vi "Main.vi"(7 "sweep rate, /min":dbl=0.2, 8 "sweep to:":dbl=-0.5, 9 "sweep":T6(radio)=enum."time_sweep") -> ()   [LabVIEW 2017] (continued)
                                n1009 = Number To Decimal String(number=w1251) -> (decimal integer string=w1250:string)  [unwired: 1 in]
                                n1010 = GPIB Write(0:w1250, 1:"OUTP?2") -> (6:w1256:errorcluster)  [unwired: 3 in, 1 out]
                                n1011 = GPIB Read(0:w1250, 1:3200, 3:w1256) -> (5:w1254:string)  [unwired: 2 in, 2 out]
                                n1012 = Fract/Exp String To Number(string=w1254) -> (number=w1253:dbl)  [unwired: 3 in, 1 out]
                                n1013 = Build Array (concatenate)(w1258, w1253) -> (w1257:dbl[])
                              }
                            }
                            n1014 = property on="data" class="Arr (strict)"("Value"=w1248) -> ()  [unwired: 2 in, 2 out]
                          }
                          frame #8 {
                            # "check if in-phase\nsignal on lock-in 5 \nis to be measured"
                            n1015 = property on="data" class="Arr (strict)"() -> ("Value"=w1260:dbl[])  [unwired: 2 in, 2 out]
                            n1016 = local read "SR830 5 ip"() -> (w1259:bool)
                            n1017 = case shown="True" w1259 {
                              tunnel: w1260 -> [w1262 w1271]
                              tunnel: [w1262 w1270] -> w1261
                              frame False {
                                # "we are not measuring in phase signal on lock-in 5 (SR830_5_ip)"
                              }
                              frame True {
                                # "we are  measuring lock-in 5 in phase (SR830_5_ip)"
                                n1018 = local read "SR830 5 addr"() -> (w1264:u8)
                                n1019 = Number To Decimal String(number=w1264) -> (decimal integer string=w1263:string)  [unwired: 1 in]
                                n1020 = GPIB Write(0:w1263, 1:"OUTP?1") -> (6:w1269:errorcluster)  [unwired: 3 in, 1 out]
                                n1021 = GPIB Read(0:w1263, 1:3200, 3:w1269) -> (5:w1267:string)  [unwired: 2 in, 2 out]
                                n1022 = Fract/Exp String To Number(string=w1267) -> (number=w1266:dbl)  [unwired: 3 in, 1 out]
                                n1023 = Build Array (concatenate)(w1271, w1266) -> (w1270:dbl[])
                              }
                            }
                            n1024 = property on="data" class="Arr (strict)"("Value"=w1261) -> ()  [unwired: 2 in, 2 out]
                          }
                          frame #9 {
                            # "check if out-of-phase\nsignal on lock-in 5 \nis to be measured"
                            n1025 = property on="data" class="Arr (strict)"() -> ("Value"=w1273:dbl[])  [unwired: 2 in, 2 out]
                            n1026 = local read "SR830 5 oop"() -> (w1272:bool)
                            n1027 = case shown="True" w1272 {
                              tunnel: w1273 -> [w1275 w1284]
                              tunnel: [w1275 w1283] -> w1274
                              frame False {
                                # "we are not measuring out of phase signal on lock-in 5 (SR830_5_oop)"
                              }
                              frame True {
                                # "we are  measuring lock-in 5 out of phase (SR830_5_oop)"
                                n1028 = local read "SR830 5 addr"() -> (w1277:u8)
                                n1029 = Number To Decimal String(number=w1277) -> (decimal integer string=w1276:string)  [unwired: 1 in]
                                n1030 = GPIB Write(0:w1276, 1:"OUTP?2") -> (6:w1282:errorcluster)  [unwired: 3 in, 1 out]
                                n1031 = GPIB Read(0:w1276, 1:3200, 3:w1282) -> (5:w1280:string)  [unwired: 2 in, 2 out]
                                n1032 = Fract/Exp String To Number(string=w1280) -> (number=w1279:dbl)  [unwired: 3 in, 1 out]
                                n1033 = Build Array (concatenate)(w1284, w1279) -> (w1283:dbl[])
                              }
                            }
                            n1034 = property on="data" class="Arr (strict)"("Value"=w1274) -> ()  [unwired: 2 in, 2 out]
                          }
                          frame #10 {
                            # "check if in-phase\nsignal on lock-in 6 \nis to be measured"
                            n1035 = property on="data" class="Arr (strict)"() -> ("Value"=w1286:dbl[])  [unwired: 2 in, 2 out]
                            n1036 = local read "SR830_6_ip"() -> (w1285:bool)
                            n1037 = case shown="True" w1285 {
                              tunnel: w1286 -> [w1288 w1297]
                              tunnel: [w1288 w1296] -> w1287
                              frame False {
                                # "we are not measuring in phase signal on lock-in 6 (SR830_6_ip)"
                              }
                              frame True {
                                # "we are  measuring lock-in 6 in phase (SR830_6_ip)"
                                n1038 = local read "SR830_6"() -> (w1290:u8)
                                n1039 = Number To Decimal String(number=w1290) -> (decimal integer string=w1289:string)  [unwired: 1 in]
                                n1040 = GPIB Write(0:w1289, 1:"OUTR?1") -> (6:w1295:errorcluster)  [unwired: 3 in, 1 out]
                                n1041 = GPIB Read(0:w1289, 1:3200, 3:w1295) -> (5:w1293:string)  [unwired: 2 in, 2 out]
                                n1042 = Fract/Exp String To Number(string=w1293) -> (number=w1292:dbl)  [unwired: 3 in, 1 out]
                                n1043 = Build Array (concatenate)(w1297, w1292) -> (w1296:dbl[])
                              }
                            }
                            n1044 = property on="data" class="Arr (strict)"("Value"=w1287) -> ()  [unwired: 2 in, 2 out]
                          }
                          frame #11 {
                            # "check if out-of-phase\nsignal on lock-in 6 \nis to be measured"
                            n1045 = property on="data" class="Arr (strict)"() -> ("Value"=w1299:dbl[])  [unwired: 2 in, 2 out]
                            n1046 = local read "SR830_6_oop"() -> (w1298:bool)
                            n1047 = case shown="True" w1298 {
                              tunnel: w1299 -> [w1301 w1310]
                              tunnel: [w1301 w1309] -> w1300
                              frame False {
                                # "we are not measuring out of phase signal on lock-in 6 (SR830_6_oop)"
                              }
                              frame True {
                                # "we are  measuring lock-in 6, out of phase (SR830_6_oop)"
                                n1048 = local read "SR830_6"() -> (w1303:u8)
                                n1049 = Number To Decimal String(number=w1303) -> (decimal integer string=w1302:string)  [unwired: 1 in]
                                n1050 = GPIB Write(0:w1302, 1:"OUTR?2") -> (6:w1308:errorcluster)  [unwired: 3 in, 1 out]
                                n1051 = GPIB Read(0:w1302, 1:3200, 3:w1308) -> (5:w1306:string)  [unwired: 2 in, 2 out]
                                n1052 = Fract/Exp String To Number(string=w1306) -> (number=w1305:dbl)  [unwired: 3 in, 1 out]
                                n1053 = Build Array (concatenate)(w1310, w1305) -> (w1309:dbl[])
                              }
                            }
                            n1054 = property on="data" class="Arr (strict)"("Value"=w1300) -> ()  [unwired: 2 in, 2 out]
                          }
                          frame #12 {
                            # "check if in-phase\nsignal on lock-in 7 \nis to be measured"
                            n1055 = property on="data" class="Arr (strict)"() -> ("Value"=w1312:dbl[])  [unwired: 2 in, 2 out]
                            n1056 = local read "SR830_7_ip"() -> (w1311:bool)
                            n1057 = case shown="True" w1311 {
                              tunnel: w1312 -> [w1314 w1323]
                              tunnel: [w1314 w1322] -> w1313
                              frame False {
                              }
                              frame True {
                                # "we are  measuring lock-in 7 in phase (SR830_7_ip)"
                                n1058 = local read "SR830_7"() -> (w1316:u8)
                                n1059 = Number To Decimal String(number=w1316) -> (decimal integer string=w1315:string)  [unwired: 1 in]
                                n1060 = GPIB Write(0:w1315, 1:"OUTR?1") -> (6:w1321:errorcluster)  [unwired: 3 in, 1 out]
                                n1061 = GPIB Read(0:w1315, 1:3200, 3:w1321) -> (5:w1319:string)  [unwired: 2 in, 2 out]
                                n1062 = Fract/Exp String To Number(string=w1319) -> (number=w1318:dbl)  [unwired: 3 in, 1 out]
                                n1063 = Build Array (concatenate)(w1323, w1318) -> (w1322:dbl[])
                              }
                            }
                            n1064 = property on="data" class="Arr (strict)"("Value"=w1313) -> ()  [unwired: 2 in, 2 out]
                          }
                          frame #13 {
                            # "check if out-of-phase\nsignal on lock-in 7 \nis to be measured"
                            n1065 = property on="data" class="Arr (strict)"() -> ("Value"=w1325:dbl[])  [unwired: 2 in, 2 out]
                            n1066 = local read "SR830_7_oop"() -> (w1324:bool)
                            n1067 = case shown="True" w1324 {
                              tunnel: w1325 -> [w1327 w1336]
                              tunnel: [w1327 w1335] -> w1326
                              frame False {
                              }
                              frame True {
                                # "we are  measuring lock-in 7 out of phase (SR830_7_oop)"
                                n1068 = local read "SR830_7"() -> (w1329:u8)
                                n1069 = Number To Decimal String(number=w1329) -> (decimal integer string=w1328:string)  [unwired: 1 in]
                                n1070 = GPIB Write(0:w1328, 1:"OUTR?2") -> (6:w1334:errorcluster)  [unwired: 3 in, 1 out]
                                n1071 = GPIB Read(0:w1328, 1:3200, 3:w1334) -> (5:w1332:string)  [unwired: 2 in, 2 out]
                                n1072 = Fract/Exp String To Number(string=w1332) -> (number=w1331:dbl)  [unwired: 3 in, 1 out]
                                n1073 = Build Array (concatenate)(w1336, w1331) -> (w1335:dbl[])
                              }
                            }
                            n1074 = property on="data" class="Arr (strict)"("Value"=w1326) -> ()  [unwired: 2 in, 2 out]
                          }
                          frame #14 {
                            # "check if in-phase\nsignal on lock-in 8 \nis to be measured"
                            n1075 = property on="data" class="Arr (strict)"() -> ("Value"=w1338:dbl[])  [unwired: 2 in, 2 out]
                            n1076 = local read "SR830_8_ip"() -> (w1337:bool)
                            n1077 = case shown="True" w1337 {
                              tunnel: w1338 -> [w1340 w1349]
                              tunnel: [w1340 w1348] -> w1339
                              frame False {
                              }
                              frame True {
                                # "we are  measuring lock-in 8 in phase (SR830_8_ip)"
                                n1078 = local read "SR830_8"() -> (w1342:u8)
                                n1079 = Number To Decimal String(number=w1342) -> (decimal integer string=w1341:string)  [unwired: 1 in]
                                n1080 = GPIB Write(0:w1341, 1:"OUTR?1") -> (6:w1347:errorcluster)  [unwired: 3 in, 1 out]
                                n1081 = GPIB Read(0:w1341, 1:3200, 3:w1347) -> (5:w1345:string)  [unwired: 2 in, 2 out]
                                n1082 = Fract/Exp String To Number(string=w1345) -> (number=w1344:dbl)  [unwired: 3 in, 1 out]
                                n1083 = Build Array (concatenate)(w1349, w1344) -> (w1348:dbl[])
                              }
                            }
                            n1084 = property on="data" class="Arr (strict)"("Value"=w1339) -> ()  [unwired: 2 in, 2 out]
                          }
                          frame #15 {
                            # "check if out-of-phase\nsignal on lock-in 8 \nis to be measured"
                            n1085 = property on="data" class="Arr (strict)"() -> ("Value"=w1351:dbl[])  [unwired: 2 in, 2 out]
                            n1086 = local read "SR830_8_oop"() -> (w1350:bool)
                            n1087 = case shown="True" w1350 {
                              tunnel: w1351 -> [w1353 w1362]
                              tunnel: [w1353 w1361] -> w1352
                              frame False {
                              }
                              frame True {
                                # "we are  measuring lock-in 8 out of phase (SR830_8_oop)"
                                n1088 = local read "SR830_8"() -> (w1355:u8)
                                n1089 = Number To Decimal String(number=w1355) -> (decimal integer string=w1354:string)  [unwired: 1 in]
                                n1090 = GPIB Write(0:w1354, 1:"OUTR?2") -> (6:w1360:errorcluster)  [unwired: 3 in, 1 out]
                                n1091 = GPIB Read(0:w1354, 1:3200, 3:w1360) -> (5:w1358:string)  [unwired: 2 in, 2 out]
                                n1092 = Fract/Exp String To Number(string=w1358) -> (number=w1357:dbl)  [unwired: 3 in, 1 out]
                                n1093 = Build Array (concatenate)(w1362, w1357) -> (w1361:dbl[])
                              }
                            }
                            n1094 = property on="data" class="Arr (strict)"("Value"=w1352) -> ()  [unwired: 2 in, 2 out]
                          }
                          frame #16 {
                            # "Measure MFLI_V if \nit is checked"
                            n1095 = property on="MFLI_V1" class="Bool (strict)"() -> ("Value"=w1363:bool)  [unwired: 2 in, 2 out]
                            n1096 = property on="data" class="Arr (strict)"() -> ("Value"=w1365:dbl[])  [unwired: 2 in, 2 out]
                            n1097 = case shown="True" w1363 {
                              tunnel: w1365 -> [w1366 w1371]
                              tunnel: [w1366 w1370] -> w1364
                              frame False {
                                # "We are not recording Step Value if it is linetrace"
                              }
                              frame True {
                                n1098 = flat-sequence {
                                tunnel: [w1375] -> w1369
                                tunnel: [w1374] -> w1368
                                tunnel: [w1373] -> w1367
                                frame #0 {
                                n1099 = property on="HandleOut" class="Clust (strict)"() -> ("Value"=w1377:T5)  [unwired: 2 in, 2 out]
                                n1100 = call "MFLIcontrol.vi"("MFLI function"=MFLIcommand."measure XY on demod0", "handle in"=w1377) -> ("Demod Sample Out 2"=w1372:T22)  [unwired: 6 in, 3 out]
                                n1101 = Unbundle(w1372) -> ("X (Vrms)"=w1375:dbl, "Y (Vrms)"=w1374:dbl, "Freq (Hz)"=w1373:dbl)  [unwired: 6 out]
                                }
                                }
                                n1102 = Build Array (concatenate)(w1371, w1369, w1368, w1367) -> (w1370:dbl[])
                              }
                            }
                            n1103 = property on="data" class="Arr (strict)"("Value"=w1364) -> ()  [unwired: 2 in, 2 out]
                          }
                          frame #17 {
                            # "Measure MFLI_I if \nit is checked"
                            n1104 = property on="MFLI_I1" class="Bool (strict)"() -> ("Value"=w1378:bool)  [unwired: 2 in, 2 out]
                            n1105 = property on="data" class="Arr (strict)"() -> ("Value"=w1380:dbl[])  [unwired: 2 in, 2 out]
                            n1106 = case shown="True" w1378 {
                              tunnel: w1380 -> [w1381 w1386]
                              tunnel: [w1381 w1385] -> w1379
                              frame False {
                                # "We are not recording Step Value if it is linetrace"
                              }
                              frame True {
                                n1107 = flat-sequence {
                                tunnel: [w1389] -> w1384
                                tunnel: [w1388] -> w1383
                                tunnel: [w1387] -> w1382
                                frame #0 {
                                n1108 = property on="HandleOut" class="Clust (strict)"() -> ("Value"=w1392:T5)  [unwired: 2 in, 2 out]
                                n1109 = call "MFLIcontrol.vi"("MFLI function"=MFLIcommand."measure current", "handle in"=w1392) -> ("Demod Sample Out 3"=w1390:T22)  [unwired: 6 in, 3 out]
                                n1110 = Unbundle(w1390) -> ("X (Vrms)"=w1389:dbl, "Y (Vrms)"=w1388:dbl, "Freq (Hz)"=w1387:dbl)  [unwired: 6 out]
                                }
                                }
                                n1111 = Build Array (concatenate)(w1386, w1384, w1383, w1382) -> (w1385:dbl[])
                              }
                            }
                            n1112 = property on="data" class="Arr (strict)"("Value"=w1379) -> ()  [unwired: 2 in, 2 out]
                          }
                          frame #18 {
                            # "Measure MFLI_V if \nit is checked"
                            n1113 = local read "MFLI_V2"() -> (w1393:bool)
                            n1114 = property on="data" class="Arr (strict)"() -> ("Value"=w1395:dbl[])  [unwired: 2 in, 2 out]
                            n1115 = case shown="True" w1393 {
                              tunnel: w1395 -> [w1396 w1401]
                              tunnel: [w1396 w1400] -> w1394
                              frame False {
                              }
                              frame True {
                                n1116 = flat-sequence {
                                tunnel: [w1406] -> w1399
                                tunnel: [w1405] -> w1398
                                tunnel: [w1404] -> w1397
                                frame #0 {
                                n1117 = property on="Handle Out 2" class="Clust (strict)"() -> ("Value"=w1402:T5)  [unwired: 2 in, 2 out]
                                n1118 = call "MFLIcontrol.vi"("MFLI function"=MFLIcommand."measure XY on demod0", "handle in"=w1402) -> ("Demod Sample Out 2"=w1403:T22)  [unwired: 6 in, 3 out]
                                n1119 = Unbundle(w1403) -> ("X (Vrms)"=w1406:dbl, "Y (Vrms)"=w1405:dbl, "Freq (Hz)"=w1404:dbl)  [unwired: 6 out]
                                }
                                }
                                n1120 = Build Array (concatenate)(w1401, w1399, w1398, w1397) -> (w1400:dbl[])
                              }
                            }
                            n1121 = property on="data" class="Arr (strict)"("Value"=w1394) -> ()  [unwired: 2 in, 2 out]
                          }
                          frame #19 {
                            # "Measure MFLI_I if \nit is checked"
                            n1122 = local read "MFLI_I2"() -> (w1408:bool)
                            n1123 = property on="data" class="Arr (strict)"() -> ("Value"=w1410:dbl[])  [unwired: 2 in, 2 out]
                            n1124 = case shown="True" w1408 {
                              tunnel: w1410 -> [w1411 w1416]
                              tunnel: [w1411 w1415] -> w1409
                              frame False {
                              }
                              frame True {
                                n1125 = flat-sequence {
                                tunnel: [w1421] -> w1414
                                tunnel: [w1420] -> w1413
                                tunnel: [w1419] -> w1412
                                frame #0 {
                                n1126 = property on="Handle Out 2" class="Clust (strict)"() -> ("Value"=w1418:T5)  [unwired: 2 in, 2 out]
                                n1127 = call "MFLIcontrol.vi"("MFLI function"=MFLIcommand."measure current", "handle in"=w1418) -> ("Demod Sample Out 3"=w1417:T22)  [unwired: 6 in, 3 out]
                                n1128 = Unbundle(w1417) -> ("X (Vrms)"=w1421:dbl, "Y (Vrms)"=w1420:dbl, "Freq (Hz)"=w1419:dbl)  [unwired: 6 out]
                                }
                                }
                                n1129 = Build Array (concatenate)(w1416, w1414, w1413, w1412) -> (w1415:dbl[])
                              }
                            }
                            n1130 = property on="data" class="Arr (strict)"("Value"=w1409) -> ()  [unwired: 2 in, 2 out]
                          }
                          frame #20 {
                            # "check if voltage \non 2400 SouceMeter 1\nis to be measured"
                            n1131 = property on="data" class="Arr (strict)"() -> ("Value"=w1424:dbl[])  [unwired: 2 in, 2 out]
                            n1132 = local read "2400 1 meas v"() -> (w1423:bool)
                            n1133 = case shown="True" w1423 {
                              tunnel: w1424 -> [w1426 w1437]
                              tunnel: [w1426 w1436] -> w1425
                              frame False {
                                # "we are not measuring 2400 1, voltage (2400_1_v)"
                              }
                              frame True {
                                # "we are  measuring 2400 1, voltage (2400_1_v)"
                                n1134 = local read "2400 1 addr"() -> (w1431:u8)
                                n1135 = Number To Decimal String(number=w1431) -> (decimal integer string=w1430:string)  [unwired: 1 in]
                                n1136 = GPIB Write(0:w1430, 1:":READ?") -> (6:w1435:errorcluster)  [unwired: 3 in, 1 out]
                                n1137 = GPIB Read(0:w1430, 1:3200, 3:w1435) -> (5:w1428:string)  [unwired: 2 in, 2 out]
                                n1138 = String Subset(string=w1428, length (rest)=13) -> (substring=w1427:string)  [unwired: 1 in]
                                n1139 = Fract/Exp String To Number(string=w1427) -> (number=w1433:dbl)  [unwired: 3 in, 1 out]
                                n1140 = Build Array (concatenate)(w1437, w1433) -> (w1436:dbl[])
                              }
                            }
                            n1141 = property on="data" class="Arr (strict)"("Value"=w1425) -> ()  [unwired: 2 in, 2 out]
                          }
                          frame #21 {
                            # "check if current \non 2400 SouceMeter 1\nis to be measured"
                            n1142 = property on="data" class="Arr (strict)"() -> ("Value"=w1439:dbl[])  [unwired: 2 in, 2 out]
                            n1143 = local read "2400 1 meas i"() -> (w1438:bool)
                            n1144 = case shown="True" w1438 {
                              tunnel: w1439 -> [w1441 w1453]
                              tunnel: [w1441 w1452] -> w1440
                              frame False {
                                # "we are not measuring 2400 1, current (2400_1_i)"
                              }
                              frame True {
                                # "we are  measuring 2400 1, current (2400_1_i)"
                                n1145 = local read "2400 1 addr"() -> (w1447:u8)
                                n1146 = Number To Decimal String(number=w1447) -> (decimal integer string=w1446:string)  [unwired: 1 in]
                                n1147 = GPIB Write(0:w1446, 1:":READ?") -> (6:w1451:errorcluster)  [unwired: 3 in, 1 out]
                                n1148 = GPIB Read(0:w1446, 1:3200, 3:w1451) -> (5:w1444:string)  [unwired: 2 in, 2 out]
                                n1149 = String Subset(string=w1444, offset (0)=14, length (rest)=13) -> (substring=w1443:string)
                                n1150 = Fract/Exp String To Number(string=w1443) -> (number=w1449:dbl)  [unwired: 3 in, 1 out]
                                n1151 = Build Array (concatenate)(w1453, w1449) -> (w1452:dbl[])
                              }
                            }
                            n1152 = property on="data" class="Arr (strict)"("Value"=w1440) -> ()  [unwired: 2 in, 2 out]
                          }
                          frame #22 {
                            # "check if voltage \non 2400 SouceMeter 2\nis to be measured"
                            n1153 = property on="data" class="Arr (strict)"() -> ("Value"=w1455:dbl[])  [unwired: 2 in, 2 out]
                            n1154 = local read "2400 2 meas v"() -> (w1454:bool)
                            n1155 = case shown="True" w1454 {
                              tunnel: w1455 -> [w1457 w1468]
                              tunnel: [w1457 w1467] -> w1456
                              frame False {
                                # "we are not measuring 2400 2, voltage (2400_2_v)"
                              }
                              frame True {
                                # "we are  measuring 2400 2, voltage (2400_2_v)"
                                n1156 = local read "2400 2 addr"() -> (w1462:u8)
                                n1157 = Number To Decimal String(number=w1462) -> (decimal integer string=w1461:string)  [unwired: 1 in]
                                n1158 = GPIB Write(0:w1461, 1:":READ?") -> (6:w1466:errorcluster)  [unwired: 3 in, 1 out]
                                n1159 = GPIB Read(0:w1461, 1:3200, 3:w1466) -> (5:w1459:string)  [unwired: 2 in, 2 out]
                                n1160 = String Subset(string=w1459, length (rest)=13) -> (substring=w1458:string)  [unwired: 1 in]
                                n1161 = Fract/Exp String To Number(string=w1458) -> (number=w1464:dbl)  [unwired: 3 in, 1 out]
                                n1162 = Build Array (concatenate)(w1468, w1464) -> (w1467:dbl[])
                              }
                            }
                            n1163 = property on="data" class="Arr (strict)"("Value"=w1456) -> ()  [unwired: 2 in, 2 out]
                          }
                          frame #23 {
                            # "check if current \non 2400 SouceMeter 2\nis to be measured"
                            n1164 = property on="data" class="Arr (strict)"() -> ("Value"=w1470:dbl[])  [unwired: 2 in, 2 out]
                            n1165 = local read "2400 2 meas i"() -> (w1469:bool)
                            n1166 = case shown="True" w1469 {
                              tunnel: w1470 -> [w1472 w1484]
                              tunnel: [w1472 w1483] -> w1471
                              frame False {
                                # "we are not measuring 2400 2, current (2400_2_i)"
                              }
                              frame True {
                                # "we are  measuring 2400 2, current (2400_2_i)"
                                n1167 = local read "2400 2 addr"() -> (w1478:u8)
                                n1168 = Number To Decimal String(number=w1478) -> (decimal integer string=w1477:string)  [unwired: 1 in]
                                n1169 = GPIB Write(0:w1477, 1:":READ?") -> (6:w1482:errorcluster)  [unwired: 3 in, 1 out]
                                n1170 = GPIB Read(0:w1477, 1:3200, 3:w1482) -> (5:w1475:string)  [unwired: 2 in, 2 out]
                                n1171 = String Subset(string=w1475, offset (0)=14, length (rest)=13) -> (substring=w1474:string)
                                n1172 = Fract/Exp String To Number(string=w1474) -> (number=w1480:dbl)  [unwired: 3 in, 1 out]
                                n1173 = Build Array (concatenate)(w1484, w1480) -> (w1483:dbl[])
                              }
                            }
                            n1174 = property on="data" class="Arr (strict)"("Value"=w1471) -> ()  [unwired: 2 in, 2 out]
                          }
                          frame #24 {
                            # "check if voltage \non 2400 SouceMeter 3\nis to be measured"
                            n1175 = property on="data" class="Arr (strict)"() -> ("Value"=w1486:dbl[])  [unwired: 2 in, 2 out]
                            n1176 = local read "2400 3 meas v"() -> (w1485:bool)
                            n1177 = case shown="True" w1485 {
                              tunnel: w1486 -> [w1488 w1499]
                              tunnel: [w1488 w1498] -> w1487
                              frame False {
                                # "we are not measuring 2400 3, voltage (2400_3_v)"
                              }
                              frame True {
                                # "we are  measuring 2400 3, voltage (2400_3_v)"
                                n1178 = local read "2400 3 addr"() -> (w1493:u8)
                                n1179 = Number To Decimal String(number=w1493) -> (decimal integer string=w1492:string)  [unwired: 1 in]
                                n1180 = GPIB Write(0:w1492, 1:":READ?") -> (6:w1497:errorcluster)  [unwired: 3 in, 1 out]
                                n1181 = GPIB Read(0:w1492, 1:3200, 3:w1497) -> (5:w1490:string)  [unwired: 2 in, 2 out]
                                n1182 = String Subset(string=w1490, length (rest)=13) -> (substring=w1489:string)  [unwired: 1 in]
                                n1183 = Fract/Exp String To Number(string=w1489) -> (number=w1495:dbl)  [unwired: 3 in, 1 out]
                                n1184 = Build Array (concatenate)(w1499, w1495) -> (w1498:dbl[])
                              }
                            }
                            n1185 = property on="data" class="Arr (strict)"("Value"=w1487) -> ()  [unwired: 2 in, 2 out]
                          }
                          frame #25 {
                            # "check if current \non 2400 SouceMeter 3\nis to be measured"
                            n1186 = property on="data" class="Arr (strict)"() -> ("Value"=w1501:dbl[])  [unwired: 2 in, 2 out]
                            n1187 = local read "2400 3 meas i"() -> (w1500:bool)
                            n1188 = case shown="True" w1500 {
                              tunnel: w1501 -> [w1503 w1515]
                              tunnel: [w1503 w1514] -> w1502
                              frame False {
                                # "we are not measuring 2400 3, current (2400_3_i)"
                              }
                              frame True {
                                # "we are  measuring 2400 3, current (2400_3_i)"
                                n1189 = local read "2400 3 addr"() -> (w1509:u8)
                                n1190 = Number To Decimal String(number=w1509) -> (decimal integer string=w1508:string)  [unwired: 1 in]
                                n1191 = GPIB Write(0:w1508, 1:":READ?") -> (6:w1513:errorcluster)  [unwired: 3 in, 1 out]
                                n1192 = GPIB Read(0:w1508, 1:3200, 3:w1513) -> (5:w1506:string)  [unwired: 2 in, 2 out]
                                n1193 = String Subset(string=w1506, offset (0)=14, length (rest)=13) -> (substring=w1505:string)
                                n1194 = Fract/Exp String To Number(string=w1505) -> (number=w1511:dbl)  [unwired: 3 in, 1 out]
                                n1195 = Build Array (concatenate)(w1515, w1511) -> (w1514:dbl[])
                              }
                            }
                            n1196 = property on="data" class="Arr (strict)"("Value"=w1502) -> ()  [unwired: 2 in, 2 out]
                          }
                          frame #26 {
                            # "check if 1st channel \non Keithley 2182A 1\nis to be measured"
                            n1197 = property on="data" class="Arr (strict)"() -> ("Value"=w1517:dbl[])  [unwired: 2 in, 2 out]
                            n1198 = local read "2182A 1 ch1"() -> (w1516:bool)
                            n1199 = case shown="True" w1516 {
                              tunnel: w1517 -> [w1519 w1528]
                              tunnel: [w1519 w1527] -> w1518
                              frame False {
                                # "we are not measuring 2182A 1 channel 1 (2182A_1_ch1)"
                              }
                              frame True {
                                # "we are  measuring 2182A 1 channel 1 (2182A_1_ch1)"
                                n1200 = local read "2182A 1 addr"() -> (w1522:u8)
                                n1201 = Number To Decimal String(number=w1522) -> (decimal integer string=w1521:string)  [unwired: 1 in]
                                n1202 = GPIB Write(0:w1521, 1:":SENSe:DATA:FRES?") -> (6:w1526:errorcluster)  [unwired: 3 in, 1 out]
                                n1203 = GPIB Read(0:w1521, 1:200, 3:w1526) -> (5:w1520:string)  [unwired: 2 in, 2 out]
                                n1204 = Fract/Exp String To Number(string=w1520) -> (number=w1524:dbl)  [unwired: 3 in, 1 out]
                                n1205 = Build Array (concatenate)(w1528, w1524) -> (w1527:dbl[])
                              }
                            }
                            n1206 = property on="data" class="Arr (strict)"("Value"=w1518) -> ()  [unwired: 2 in, 2 out]
                          }
                          frame #27 {
                            # "check if 2nd channel \non Keithley 2182A 1\nis to be measured"
                            n1207 = property on="data" class="Arr (strict)"() -> ("Value"=w1530:dbl[])  [unwired: 2 in, 2 out]
                            n1208 = local read "2182A 1 ch2"() -> (w1529:bool)
                            n1209 = case shown="True" w1529 {
                              tunnel: w1530 -> [w1532 w1545]
                              tunnel: [w1532 w1544] -> w1531
                              frame False {
                                # "we are not measuring 2182A 1 channel 2 (2182A_1_ch2)"
                              }
                              frame True {
                                # "switching to channel 2 and then\nback to channel 1"
                                # "we are  measuring 2182A 1 channel 2 (2182A_1_ch2)"
                                n1210 = local read "2182A 1 addr"() -> (w1539:u8)
                                n1211 = Number To Decimal String(number=w1539) -> (decimal integer string=w1534:string)  [unwired: 1 in]
                                n1212 = GPIB Write(0:w1534, 1:":SENSe:CHAN 2") -> (6:w1536:errorcluster)  [unwired: 3 in, 1 out]
                                n1213 = GPIB Write(0:w1534, 1:":SENSe:DATA:FRES?", 3:w1536) -> (6:w1543:errorcluster)  [unwired: 2 in, 1 out]
                                n1214 = GPIB Read(0:w1534, 1:200, 3:w1543) -> (5:w1538:string, 7:w1535:errorcluster)  [unwired: 2 in, 1 out]
                                n1215 = GPIB Write(0:w1534, 1:":SENSe:CHAN 1", 3:w1535) -> ()  [unwired: 2 in, 2 out]
                                n1216 = Fract/Exp String To Number(string=w1538) -> (number=w1541:dbl)  [unwired: 3 in, 1 out]
                                n1217 = Build Array (concatenate)(w1545, w1541) -> (w1544:dbl[])
                              }
                            }
                            n1218 = property on="data" class="Arr (strict)"("Value"=w1531) -> ()  [unwired: 2 in, 2 out]
                          }
                          frame #28 {
                            # "check if 1st channel \non Keithley 2182A 2\nis to be measured"
                            n1219 = property on="data" class="Arr (strict)"() -> ("Value"=w1547:dbl[])  [unwired: 2 in, 2 out]
                            n1220 = local read "2182A 2 ch1"() -> (w1546:bool)
                            n1221 = case shown="True" w1546 {
                              tunnel: w1547 -> [w1549 w1558]
                              tunnel: [w1549 w1557] -> w1548
                              frame False {
                                # "we are not measuring 2182A 2 channel 1 (2182A_2_ch1)"
                              }
                              frame True {
                                # "we are  measuring 2182A 2 channel 1 (2182A_2_ch1)"
                                n1222 = local read "2182A 2 addr"() -> (w1552:u8)
                                n1223 = Number To Decimal String(number=w1552) -> (decimal integer string=w1551:string)  [unwired: 1 in]
                                n1224 = GPIB Write(0:w1551, 1:":SENSe:DATA:FRES?") -> (6:w1556:errorcluster)  [unwired: 3 in, 1 out]
                                n1225 = GPIB Read(0:w1551, 1:200, 3:w1556) -> (5:w1550:string)  [unwired: 2 in, 2 out]
                                n1226 = Fract/Exp String To Number(string=w1550) -> (number=w1554:dbl)  [unwired: 3 in, 1 out]
                                n1227 = Build Array (concatenate)(w1558, w1554) -> (w1557:dbl[])
                              }
                            }
                            n1228 = property on="data" class="Arr (strict)"("Value"=w1548) -> ()  [unwired: 2 in, 2 out]
                          }
                          frame #29 {
                            # "check if 2nd channel \non Keithley 2182A 2\nis to be measured"
                            n1229 = property on="data" class="Arr (strict)"() -> ("Value"=w1560:dbl[])  [unwired: 2 in, 2 out]
                            n1230 = local read "2182A 2 ch2"() -> (w1559:bool)
                            n1231 = case shown="True" w1559 {
                              tunnel: w1560 -> [w1562 w1575]
                              tunnel: [w1562 w1574] -> w1561
                              frame False {
                                # "we are not measuring 2182A 2 channel 2 (2182A_2_ch2)"
                              }
                              frame True {
                                # "switching to channel 2 and then\nback to channel 1"
                                # "we are  measuring 2182A 2 channel 2 (2182A_2_ch2)"
                                n1232 = local read "2182A 2 addr"() -> (w1569:u8)
                                n1233 = Number To Decimal String(number=w1569) -> (decimal integer string=w1564:string)  [unwired: 1 in]
                                n1234 = GPIB Write(0:w1564, 1:":SENSe:CHAN 2") -> (6:w1566:errorcluster)  [unwired: 3 in, 1 out]
                                n1235 = GPIB Write(0:w1564, 1:":SENSe:DATA:FRES?", 3:w1566) -> (6:w1573:errorcluster)  [unwired: 2 in, 1 out]
                                n1236 = GPIB Read(0:w1564, 1:200, 3:w1573) -> (5:w1568:string, 7:w1565:errorcluster)  [unwired: 2 in, 1 out]
                                n1237 = GPIB Write(0:w1564, 1:":SENSe:CHAN 1", 3:w1565) -> ()  [unwired: 2 in, 2 out]
                                n1238 = Fract/Exp String To Number(string=w1568) -> (number=w1571:dbl)  [unwired: 3 in, 1 out]
                                n1239 = Build Array (concatenate)(w1575, w1571) -> (w1574:dbl[])
                              }
                            }
                            n1240 = property on="data" class="Arr (strict)"("Value"=w1561) -> ()  [unwired: 2 in, 2 out]
                          }
                          frame #30 {
                            # "check if 1st channel \non Keithley 2182A 3\nis to be measured"
                            n1241 = property on="data" class="Arr (strict)"() -> ("Value"=w1577:dbl[])  [unwired: 2 in, 2 out]
                            n1242 = local read "2182A 3 ch1"() -> (w1576:bool)
                            n1243 = case shown="True" w1576 {
                              tunnel: w1577 -> [w1579 w1588]
                              tunnel: [w1579 w1587] -> w1578
                              frame False {
                                # "we are not measuring 2182A 3 channel 1 (2182A_3_ch1)"
                              }
                              frame True {
                                # "we are  measuring 2182A 3 channel 1 (2182A_3_ch1)"
                                n1244 = local read "2182A 3 addr"() -> (w1582:u8)
                                n1245 = Number To Decimal String(number=w1582) -> (decimal integer string=w1581:string)  [unwired: 1 in]
                                n1246 = GPIB Write(0:w1581, 1:":SENSe:DATA:FRES?") -> (6:w1586:errorcluster)  [unwired: 3 in, 1 out]
                                n1247 = GPIB Read(0:w1581, 1:200, 3:w1586) -> (5:w1580:string)  [unwired: 2 in, 2 out]
                                n1248 = Fract/Exp String To Number(string=w1580) -> (number=w1584:dbl)  [unwired: 3 in, 1 out]
                                n1249 = Build Array (concatenate)(w1588, w1584) -> (w1587:dbl[])
                              }
                            }
                            n1250 = property on="data" class="Arr (strict)"("Value"=w1578) -> ()  [unwired: 2 in, 2 out]
                          }
                          frame #31 {
                            # "check if 2nd channel \non Keithley 2182A 3\nis to be measured"
                            n1251 = property on="data" class="Arr (strict)"() -> ("Value"=w1590:dbl[])  [unwired: 2 in, 2 out]
                            n1252 = local read "2182A 3 ch2"() -> (w1589:bool)
                            n1253 = case shown="True" w1589 {
                              tunnel: w1590 -> [w1592 w1605]
                              tunnel: [w1592 w1604] -> w1591
                              frame False {
                                # "we are not measuring 2182A 3 channel 2 (2182A_3_ch2)"
                              }
                              frame True {
                                # "switching to channel 2 and then\nback to channel 1"
                                # "we are  measuring 2182A 3 channel 2 (2182A_3_ch2)"
                                n1254 = local read "2182A 3 addr"() -> (w1599:u8)
                                n1255 = Number To Decimal String(number=w1599) -> (decimal integer string=w1594:string)  [unwired: 1 in]
                                n1256 = GPIB Write(0:w1594, 1:":SENSe:CHAN 2") -> (6:w1596:errorcluster)  [unwired: 3 in, 1 out]
                                n1257 = GPIB Write(0:w1594, 1:":SENSe:DATA:FRES?", 3:w1596) -> (6:w1603:errorcluster)  [unwired: 2 in, 1 out]
                                n1258 = GPIB Read(0:w1594, 1:200, 3:w1603) -> (5:w1598:string, 7:w1595:errorcluster)  [unwired: 2 in, 1 out]
                                n1259 = GPIB Write(0:w1594, 1:":SENSe:CHAN 1", 3:w1595) -> ()  [unwired: 2 in, 2 out]
                                n1260 = Fract/Exp String To Number(string=w1598) -> (number=w1601:dbl)  [unwired: 3 in, 1 out]
                                n1261 = Build Array (concatenate)(w1605, w1601) -> (w1604:dbl[])
                              }
                            }
                            n1262 = property on="data" class="Arr (strict)"("Value"=w1591) -> ()  [unwired: 2 in, 2 out]
                          }
                          frame #32 {
                            # "check if 1st channel \non Keithley 2182A 4\nis to be measured"
                            n1263 = property on="data" class="Arr (strict)"() -> ("Value"=w1607:dbl[])  [unwired: 2 in, 2 out]
                            n1264 = local read "2182A 4 ch1"() -> (w1606:bool)
                            n1265 = case shown="True" w1606 {
                              tunnel: w1607 -> [w1609 w1618]
                              tunnel: [w1609 w1617] -> w1608
                              frame False {
                                # "we are not measuring 2182A 4 channel 1 (2182A_4_ch1)"
                              }
                              frame True {
                                # "we are  measuring 2182A 4 channel 1 (2182A_4_ch1)"
                                n1266 = local read "2182A 4 addr"() -> (w1612:u8)
                                n1267 = Number To Decimal String(number=w1612) -> (decimal integer string=w1611:string)  [unwired: 1 in]
                                n1268 = GPIB Write(0:w1611, 1:":SENSe:DATA:FRES?") -> (6:w1616:errorcluster)  [unwired: 3 in, 1 out]
                                n1269 = GPIB Read(0:w1611, 1:200, 3:w1616) -> (5:w1610:string)  [unwired: 2 in, 2 out]
                                n1270 = Fract/Exp String To Number(string=w1610) -> (number=w1614:dbl)  [unwired: 3 in, 1 out]
                                n1271 = Build Array (concatenate)(w1618, w1614) -> (w1617:dbl[])
                              }
                            }
                            n1272 = property on="data" class="Arr (strict)"("Value"=w1608) -> ()  [unwired: 2 in, 2 out]
                          }
                          frame #33 {
                            # "check if 2nd channel \non Keithley 2182A 4\nis to be measured"
                            n1273 = property on="data" class="Arr (strict)"() -> ("Value"=w1620:dbl[])  [unwired: 2 in, 2 out]
                            n1274 = local read "2182A 4 ch2"() -> (w1619:bool)
                            n1275 = case shown="False" w1619 {
                              tunnel: w1620 -> [w1622 w1635]
                              tunnel: [w1622 w1634] -> w1621
                              frame False {
                                # "we are not measuring 2182A 4 channel 2 (2182A_4_ch2)"
                              }
                              frame True {
                                # "switching to channel 2 and then\nback to channel 1"
                                # "we are  measuring 2182A 4 channel 2 (2182A_4_ch2)"
                                n1276 = local read "2182A 4 addr"() -> (w1629:u8)
                                n1277 = Number To Decimal String(number=w1629) -> (decimal integer string=w1624:string)  [unwired: 1 in]
                                n1278 = GPIB Write(0:w1624, 1:":SENSe:CHAN 2") -> (6:w1626:errorcluster)  [unwired: 3 in, 1 out]
                                n1279 = GPIB Write(0:w1624, 1:":SENSe:DATA:FRES?", 3:w1626) -> (6:w1633:errorcluster)  [unwired: 2 in, 1 out]
                                n1280 = GPIB Read(0:w1624, 1:200, 3:w1633) -> (5:w1628:string, 7:w1625:errorcluster)  [unwired: 2 in, 1 out]
                                n1281 = GPIB Write(0:w1624, 1:":SENSe:CHAN 1", 3:w1625) -> ()  [unwired: 2 in, 2 out]
                                n1282 = Fract/Exp String To Number(string=w1628) -> (number=w1631:dbl)  [unwired: 3 in, 1 out]
                                n1283 = Build Array (concatenate)(w1635, w1631) -> (w1634:dbl[])
                              }
                            }
                            n1284 = property on="data" class="Arr (strict)"("Value"=w1621) -> ()  [unwired: 2 in, 2 out]
                          }
                          frame #34 {
                            # "check if voltage on\nKeithley 2636A smua\nis to be measured"
                            n1285 = local read "2636A smua meas v"() -> (w1636:bool)
                            n1286 = property on="data" class="Arr (strict)"() -> ("Value"=w1637:dbl[])  [unwired: 2 in, 2 out]
                            n1287 = case shown="True" w1636 {
                              tunnel: w1637 -> [w1639 w1645]
                              tunnel: [w1639 w1644] -> w1638
                              frame False {
                                # "we are not measuring voltage on 2636A smua (2636A_smua_v)"
                              }
                              frame True {
                                # "we are  measuring voltage on 2636A smua (2636A_smua_v)"
                                n1288 = local read "2336A addr"() -> (w1640:refnum<visa-resource-name>)
                                n1289 = call "SinglePointMeasurement.vi"("Measure"=Measure."Voltage", "Channel"=Channel."a", "VISA resource name 2"=w1640) -> ("Measuremet"=w1642:dbl)  [unwired: 3 in, 4 out]
                                n1290 = Build Array (concatenate)(w1645, w1642) -> (w1644:dbl[])
                              }
                            }
                            n1291 = property on="data" class="Arr (strict)"("Value"=w1638) -> ()  [unwired: 2 in, 2 out]
                          }
                          frame #35 {
                            # "check if current on\nKeithley 2636A smua\nis to be measured"
                            n1292 = local read "2636A smua meas i"() -> (w1646:bool)
                            n1293 = property on="data" class="Arr (strict)"() -> ("Value"=w1647:dbl[])  [unwired: 2 in, 2 out]
                            n1294 = case shown="True" w1646 {
                              tunnel: w1647 -> [w1649 w1652]
                              tunnel: [w1649 w1651] -> w1648
                              frame False {
                                # "we are not measuring current on 2636A smua (2636A_smua_i)"
                              }
                              frame True {
                                # "we are  measuring current on 2636A smua (2636A_smua_i)"
                                n1295 = stacked-sequence {
                                tunnel: [_ w1661] -> w1650
                                frame #0 {
                                n1296 = local read "auto\nrange A"() -> (w1656:bool)
                                n1297 = local read "2336A addr"() -> (w1659:refnum<visa-resource-name>)
                                n1298 = Select(t="smua.AUTORANGE_ON", s=w1656, f="smua.AUTORANGE_OFF") -> (s? t:f=w1654:string)
                                n1299 = Concatenate Strings("smua.measure.autorangei = ", w1654) -> (w1653:string)
                                n1300 = VISA Write(VISA resource name=w1659, write buffer=w1653) -> ()  [unwired: 1 in, 3 out]
                                }
                                frame #1 {
                                n1301 = local read "2336A addr"() -> (w1663:refnum<visa-resource-name>)
                                n1302 = call "SinglePointMeasurement.vi"("Measure"=Measure."Current", "Channel"=Channel."a", "VISA resource name 2"=w1663) -> ("Measuremet"=w1661:dbl)  [unwired: 3 in, 4 out]
                                }
                                }
                                n1303 = Build Array (concatenate)(w1652, w1650) -> (w1651:dbl[])
                              }
                            }
                            n1304 = property on="data" class="Arr (strict)"("Value"=w1648) -> ()  [unwired: 2 in, 2 out]
                          }
                          frame #36 {
                            # "check if voltage on\nKeithley 2636A smub\nis to be measured"
                            n1305 = local read "2636A smub meas v"() -> (w1664:bool)
                            n1306 = property on="data" class="Arr (strict)"() -> ("Value"=w1665:dbl[])  [unwired: 2 in, 2 out]
                            n1307 = case shown="True" w1664 {
                              tunnel: w1665 -> [w1667 w1673]
                              tunnel: [w1667 w1672] -> w1666
                              frame False {
                                # "we are not measuring voltage on 2636A smub (2636A_smub_v)"
                              }
                              frame True {
                                # "we are  measuring voltage on 2636A smub (2636A_smub_v)"
                                n1308 = local read "2336A addr"() -> (w1671:refnum<visa-resource-name>)
                                n1309 = call "SinglePointMeasurement.vi"("Measure"=Measure."Voltage", "Channel"=Channel."b", "VISA resource name 2"=w1671) -> ("Measuremet"=w1669:dbl)  [unwired: 3 in, 4 out]
                                n1310 = Build Array (concatenate)(w1673, w1669) -> (w1672:dbl[])
                              }
                            }
                            n1311 = property on="data" class="Arr (strict)"("Value"=w1666) -> ()  [unwired: 2 in, 2 out]
                          }
                          frame #37 {
                            # "check if current on\nKeithley 2636A smub\nis to be measured"
                            n1312 = local read "2636A smub meas i"() -> (w1674:bool)
                            n1313 = property on="data" class="Arr (strict)"() -> ("Value"=w1675:dbl[])  [unwired: 2 in, 2 out]
                            n1314 = case shown="True" w1674 {
                              tunnel: w1675 -> [w1677 w1680]
                              tunnel: [w1677 w1679] -> w1676
                              frame False {
                                # "we are not measuring current on 2636A smub (2636A_smub_i)"
                              }
                              frame True {
                                # "we are  measuring current on 2636A smub (2636A_smub_i)"
                                n1315 = stacked-sequence {
                                tunnel: [_ w1689] -> w1678
                                frame #0 {
                                n1316 = local read "auto\nrange B"() -> (w1684:bool)
                                n1317 = local read "2336A addr"() -> (w1687:refnum<visa-resource-name>)
                                n1318 = Select(t="smub.AUTORANGE_ON", s=w1684, f="smub.AUTORANGE_OFF") -> (s? t:f=w1682:string)
                                n1319 = Concatenate Strings("smub.measure.autorangei = ", w1682) -> (w1681:string)
                                n1320 = VISA Write(VISA resource name=w1687, write buffer=w1681) -> ()  [unwired: 1 in, 3 out]
                                }
                                frame #1 {
                                n1321 = local read "2336A addr"() -> (w1691:refnum<visa-resource-name>)
                                n1322 = call "SinglePointMeasurement.vi"("Measure"=Measure."Current", "Channel"=Channel."b", "VISA resource name 2"=w1691) -> ("Measuremet"=w1689:dbl)  [unwired: 3 in, 4 out]
                                }
                                }
                                n1323 = Build Array (concatenate)(w1680, w1678) -> (w1679:dbl[])
                              }
                            }
                            n1324 = property on="data" class="Arr (strict)"("Value"=w1676) -> ()  [unwired: 2 in, 2 out]
                          }
                          frame #38 {
                            # "check if time\nis to be measured"
                            n1325 = property on="data" class="Arr (strict)"() -> ("Value"=w1693:dbl[])  [unwired: 2 in, 2 out]
                            n1326 = local read "measure time"() -> (w1692:bool)
                            n1327 = case shown="True" w1692 {
                              tunnel: w1693 -> [w1695 w1701]
                              tunnel: [w1695 w1700] -> w1694
                              frame False {
                                # "we are not measuring time"
                              }
                              frame True {
                                # "seconds from the beginning of month"
                                # "we are  measuring time"
                                n1328 = call "timeInSeconds.vi"() -> ("Numeric"=w1699:dbl, "current time"=w1697:timestamp)  [unwired: 2 in]
                                n1329 = property on="current time" class="AbsTime (strict)"("Value"=w1697) -> ()  [unwired: 2 in, 2 out]
                                n1330 = Subtract(x=w1699, y=0.0) -> (x-y=w1698:dbl)
                                n1331 = Build Array (concatenate)(w1701, w1698) -> (w1700:dbl[])
                              }
                            }
                            n1332 = property on="data" class="Arr (strict)"("Value"=w1694) -> ()  [unwired: 2 in, 2 out]
                          }
                          frame #39 {
                            n1333 = local read "iPS_MagnetField"() -> (w1702:bool)
                            n1334 = property on="data" class="Arr (strict)"() -> ("Value"=w1703:dbl[])  [unwired: 2 in, 2 out]
                            n1335 = case shown="True" w1702 {
                              tunnel: w1703 -> [w1705 w1710]
                              tunnel: [w1705 w1709] -> w1704
                              frame False {
                                # "we are not Measuring magnetic field on IPS120-0"
                              }
                              frame True {
                                # "Measure magnetic field on Teslatron_iPS_Field"
                                n1336 = local read "iPS_addr_sweep"() -> (w1708:refnum<visa-resource-name>)
                                n1337 = call "iPSread.vi"("iPSreadCtrl"=iPSreadCtrl."MagnetField", "VISA resource name"=w1708) -> ("number"=w1707:dbl)  [unwired: 6 in, 3 out]
                                n1338 = Build Array (concatenate)(w1710, w1707) -> (w1709:dbl[])
                              }
                            }
                            n1339 = property on="data" class="Arr (strict)"("Value"=w1704) -> ()  [unwired: 2 in, 2 out]
                          }
                          frame #40 {
                            n1340 = property on="data" class="Arr (strict)"() -> ("Value"=w1712:dbl[])  [unwired: 2 in, 2 out]
                            n1341 = property on="Magnet_T" class="Bool (strict)"() -> ("Value"=w1711:bool)  [unwired: 2 in, 2 out]
                            n1342 = case shown="True" w1711 {
                              tunnel: w1712 -> [w1714 w1719]
                              tunnel: [w1714 w1718] -> w1713
                              frame False {
                                # "we are not Measuring magnetic field on IPS120-0"
                              }
                              frame True {
                                # "Measure magnetic_T on Teslatron"
                                n1343 = local read "iPS_addr_sweep"() -> (w1717:refnum<visa-resource-name>)
                                n1344 = call "iPSread.vi"("iPSreadCtrl"=iPSreadCtrl."Magnet Temp", "VISA resource name"=w1717) -> ("number"=w1716:dbl)  [unwired: 6 in, 3 out]
                                n1345 = Build Array (concatenate)(w1719, w1716) -> (w1718:dbl[])
                              }
                            }
                            n1346 = property on="data" class="Arr (strict)"("Value"=w1713) -> ()  [unwired: 2 in, 2 out]
                          }
                          frame #41 {
                            n1347 = property on="data" class="Arr (strict)"() -> ("Value"=w1721:dbl[])  [unwired: 2 in, 2 out]
                            n1348 = property on="SH_T" class="Bool (strict)"() -> ("Value"=w1720:bool)  [unwired: 2 in, 2 out]
                            n1349 = case shown="True" w1720 {
                              tunnel: w1721 -> [w1723 w1728]
                              tunnel: [w1723 w1727] -> w1722
                              frame False {
                                # "we are not Measuring magnetic field on IPS120-0"
                              }
                              frame True {
                                # "Measure  SH_T on Teslatron"
                                n1350 = local read "iPS_addr_sweep"() -> (w1726:refnum<visa-resource-name>)
                                n1351 = call "iPSread.vi"("iPSreadCtrl"=iPSreadCtrl."Switch Heater Temp", "VISA resource name"=w1726) -> ("number"=w1725:dbl)  [unwired: 6 in, 3 out]
                                n1352 = Build Array (concatenate)(w1728, w1725) -> (w1727:dbl[])
                              }
                            }
